vi "check vid path.vi"(9 "Trial #":u32, 10 "Experiment Name":string, 11 "Data Output Directory":path) -> (3 "appended path":path)   [LabVIEW 2019]
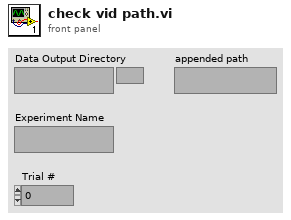
[diagram p1: front panel]
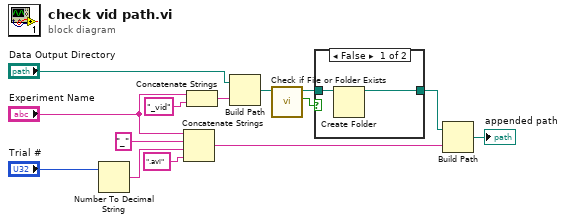
[diagram p0: block diagram]
diagram:
  n1 = Number To Decimal String(number="Trial #") -> (decimal integer string=w10:string)  [unwired: 1 in]
  n2 = Concatenate Strings("Experiment Name", "_" ("string"), w10, ".avi" ("string")) -> (w12:string)
  n3 = Concatenate Strings("Experiment Name", "_vid" ("string")) -> (w5:string)
  n4 = Build Path(base path="Data Output Directory", name or relative path=w5) -> (appended path=w4:path)
  n5 = call <vilib>:"Check if File or Folder Exists.vi"("path"=w4) -> ("file or folder exists?"=w14:bool, "dup path"=w3:path)  [unwired: 8 in, 1 out]
  n6 = case shown="False" w14 {
    tunnel: w3 -> [w16 w17]
    tunnel: [w15 w17] -> w13
    frame False {
      n7 = Create Folder(path (use dialog)=w16) -> (created path=w15:path)  [unwired: 2 in, 2 out]
    }
    frame True {
    }
  }
  n8 = Build Path(base path=w13, name or relative path=w12) -> (appended path=→"appended path":path)
